vi "Close Group.vi"(8 "error in (no error)":errorcluster, 11 "group_id":i32) -> (0 "error out":errorcluster)   [LabVIEW 2010, in "HDF5Tools.lvlib"]
uses:
  HDF5Tools.lvlib
  Release/HDF5Tools.dll
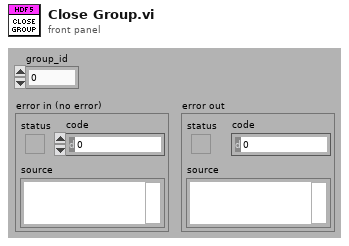
[diagram p1: front panel]
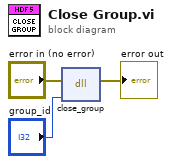
[diagram p0: block diagram]
diagram:
  n1 = dll-call lib="Z:/libraries/HDF5Tools/Release/HDF5Tools.dll" fn="close_group"(error in="error in (no error)", "group_id"="group_id") -> (error out=→"error out":errorcluster)  [unwired: 4 in, 1 out]
